vi "Read commandStart.vi"(8 "error in (no error)":errorcluster, 11 "SettingUpState in":refnum<class "SettingUpState.lvclass">) -> (0 "error out":errorcluster, 2 "commandStart":dbl, 3 "SettingUpState out":refnum<class "SettingUpState.lvclass">)   [LabVIEW 2020, in "SettingUpState.lvclass"]
uses:
  SettingUpState.lvclass
  SettingUpState.lvclass/SettingUpState.ctl
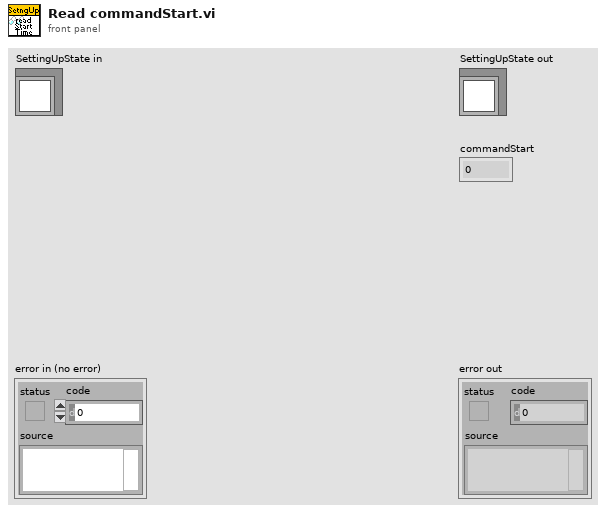
[diagram p1: front panel]
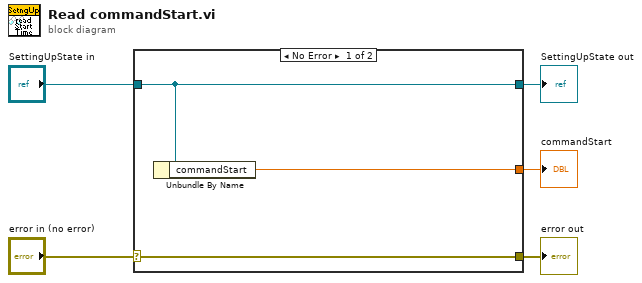
[diagram p0: block diagram]
diagram:
  n1 = case shown="No Error" "error in (no error)" {
    selector: "error in (no error)" -> [w8 w9]
    tunnel: [w8 w9] -> w4
    tunnel: [w7 w10] -> w2
    tunnel: "SettingUpState in" -> [w7 w10]
    tunnel: [w6 _] -> w1
    frame No Error {
      n2 = Unbundle By Name(w7) -> ("commandStart"=w6:dbl)
    }
    frame Error {
    }
  }
  "error out" <- w4
  "SettingUpState out" <- w2
  "commandStart" <- w1
